vi "LVClass_HasoData Get ProcessorList.vi"(0 "HasoData in":refnum<class "HasoData.lvclass">, 5 "SlopesPostProcessorList in":refnum<class "SlopesPostProcessorList.lvclass">, 11 "error in (no error)":errorcluster) -> (4 "HasoData out":refnum<class "HasoData.lvclass">, 6 "SlopesPostProcessorList out":refnum<class "SlopesPostProcessorList.lvclass">, 15 "error out":errorcluster)   [LabVIEW 2020, in "HasoData.lvclass"]
doc: "SlopesPostProcessorList getter.\n\n--------------------------------------------------------------------------------\n\n<B>HasoDataIn</B> : HasoData object.\n<B>HasoDataOut</B> : HasoData object.\n<B>SlopesPostProcessorList in</B> : SlopesPostProcessorList object to store the SlopesPostProcessorList \n<B>SlopesPostProcessorList out</B> : SlopesPostProcessorList object upadted with the current SlopesPostProcessorList\n\n\n--------------------------------------------------------------------------------"
uses:
  HasoData.lvclass
  SlopesPostProcessorList/SlopesPostProcessorList.lvclass
  HasoData.lvclass/HasoData.ctl
  SlopesPostProcessorList/LVClass_SlopesPostProcessList Read SlopesPostProccessor.vi
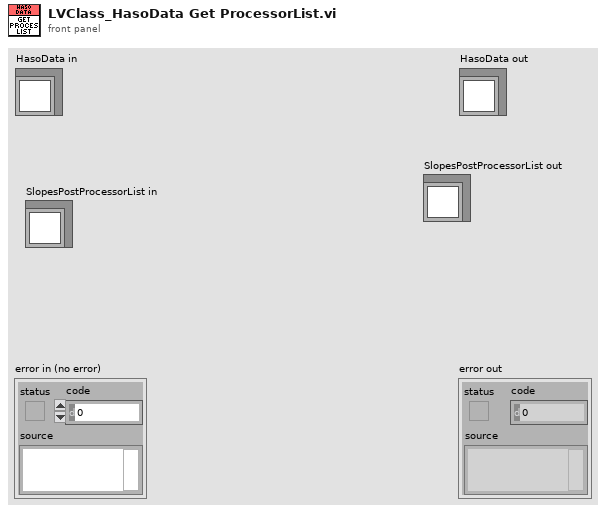
[diagram p1: front panel]
types:
  T1 = typedef "ClassID.ctl" = i64
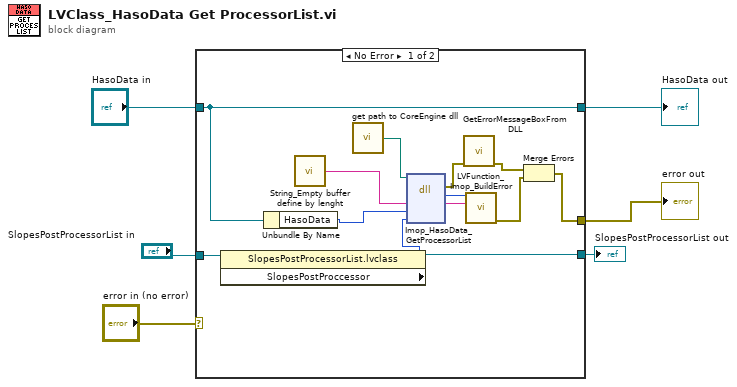
[diagram p0: block diagram]
diagram:
  n1 = case shown="No Error" "error in (no error)" {
    selector: "error in (no error)" -> [_ w22]
    tunnel: [w7 w22] -> w4
    tunnel: [w12 w21] -> w3
    tunnel: "HasoData in" -> [w12 w21]
    tunnel: "SlopesPostProcessorList in" -> [w14 w20]
    tunnel: [w10 w20] -> w1
    frame No Error {
      n2 = property class="SlopesPostProcessorList.lvclass"(reference=w14) -> (reference out=w10:refnum<class "SlopesPostProcessorList.lvclass">, "SlopesPostProccessor"=w13:T1)  [unwired: 1 in, 1 out]
      n3 = Unbundle By Name(w12) -> ("HasoData"=w11:T1)
      n4 = call "String_Empty buffer define by lenght.vi"() -> ("Empty buffer"=w17:string)  [unwired: 1 in]
      n5 = call "get path to CoreEngine dll.vi"() -> ("path to wavekit library"=w16:path)  [unwired: 14 in, 1 out]
      n6 = dll-call lib="D:/2_trunk/Soft_haso/ImOpCoreEngine4_LV2011/DLLs/ImopEngine4_vc100.dll" fn="Imop_HasoData_GetProcessorList"(path in=w16, "message"=w17, "objet"=w11, "List"=w13) -> (error out=w15:errorcluster, "return type"=w19:i32, "message"=w18:string)  [unwired: 4 in, 1 out]
      n7 = call "GetErrorMessageBoxFromDLL.vi"("error IN"=w15) -> ("error OUT"=w9:errorcluster)  [unwired: 10 in]
      n8 = call "LVFunction_Imop_BuildError.vi"("code"=w19, "String to Prepend to source (\"\")"=w18) -> ("error out"=w8:errorcluster)  [unwired: 13 in]
      n9 = Merge Errors(w9, w8) -> (w7:errorcluster)
    }
    frame Error {
    }
  }
  "error out" <- w4
  "HasoData out" <- w3
  "SlopesPostProcessorList out" <- w1
